vi "Close.vi"(8 "error in (no error)":errorcluster, 11 "VISA resource name":refnum<visa-resource-name>) -> (0 "error out":errorcluster)   [LabVIEW 2017]
doc: "Interrupt current motion.\nQuit onl-line mode and return to Local mode.\nClose VISA session."
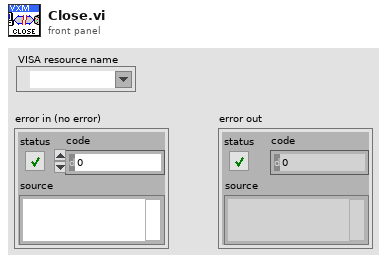
[diagram p1: front panel]
types:
  T1 = enum16{"Cmd-Response", "Write Only", "Read Only"}
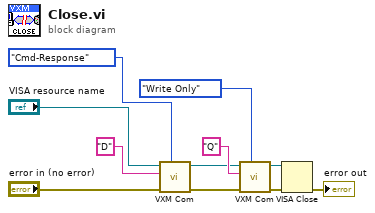
[diagram p0: block diagram]
diagram:
  n1 = call "VXM Com.vi"("Operation"=T1."Cmd-Response", "error in (no error)"="error in (no error)", "Write Buffer ('/' codes)"="D" ("Write Buffer"), "VISA resource name"="VISA resource name") -> ("error out"=w6:errorcluster, "VISA resource out"=w7:refnum<visa-resource-name>)  [unwired: 5 in, 1 out]
  n2 = call "VXM Com.vi"("Operation"=T1."Write Only", "error in (no error)"=w6, "Write Buffer ('/' codes)"="Q" ("Write Buffer"), "VISA resource name"=w7) -> ("error out"=w4:errorcluster, "VISA resource out"=w5:refnum<visa-resource-name>)  [unwired: 5 in, 1 out]
  n3 = VISA Close(VISA resource name=w5, error in (no error)=w4) -> (error out=→"error out":errorcluster)
